vi "get target editor class.vi"(8 "error in":errorcluster, 11 "TBM Configuration":refnum<class "TBM configuration.lvclass">) -> (0 "error out":errorcluster, 2 "class name":string)   [LabVIEW 2013, in "PL Framework Configuration Tool.lvlib" / "Targets.lvclass"]
uses:
  Targets.lvclass
  <vilib>/NI/Tag Bus Module Framework/root configuration/TBM configuration.lvclass
  Framework Configuration Classes/target configuration/PL_Target Configuration.lvclass
  Framework Configuration Classes/target configuration/PL_Target Configuration.lvclass/PL_Target Configuration.ctl
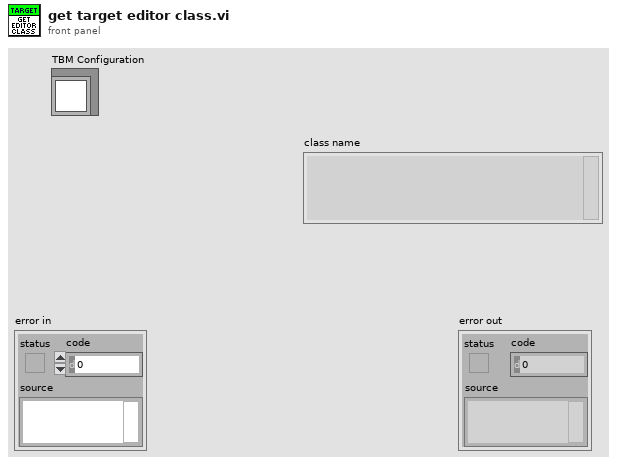
[diagram p1: front panel]
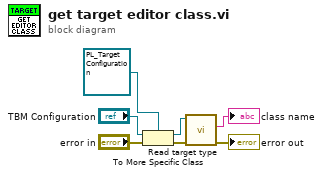
[diagram p0: block diagram]
diagram:
  n1 = To More Specific Class(target class=refnum<class "PL_Target Configuration.lvclass"> refnum ("Target Configuration"), reference="TBM Configuration", error in="error in") -> (specific class reference=w5:refnum<class "PL_Target Configuration.lvclass">, error out=w1:errorcluster)
  n2 = call "Read target type.vi"("error in"=w1, "PL_Target Configuration in"=w5) -> ("error out"=→"error out":errorcluster, "hardware class"=→"class name":string)  [unwired: 7 in, 1 out]
